vi "SynchIO.MyTest.vi"() -> ()   [LabVIEW 2016, in "SynchIO.lvclass"]
doc: "JKI State Machine Objects (SMO) 1.0.0.5\nJKI - JKI\nCopyright (c) 2016, JKI"
uses:
  SynchIO.lvclass
  C:/Program Files (x86)/National Instruments/LabVIEW 2016/vi.lib/JKI/JKI SMO/SMO/SMO.lvclass
  SynchIO.USB4431/SynchIO.USB4431.lvclass
  I:/levy_SVN/lockin/branches/jlevy/SMO/SynchIO/SynchIO.lvclass
  <vilib>/JKI/JKI SMO/SMO/Typedefs/SMOState --Enum.ctl
  <vilib>/JKI/JKI SMO/SMO/SMO.lvclass
panel:
  out "Input Signals":waveform(dbl)[](array[waveform])
  in  "4431?":bool=TRUE
  in  "IO Info":T1={"AI task"=["ai", ""], "sampling info"={"Fs"=1000.0, "#s"=1000.0}, "AO Array"=[], "AO Task"=["ao"], "Reset"=FALSE} {"sampling info"."Fs" format="%.2p"}
  out "Old Value":string
  out "New Value":string
  in  "Send":bool
  in  "Data":string
  out "error out":errorcluster
  in  "Stop":bool
  # "For instructions on how to use the JKI State Machine Objects, examples and video tutorials, visit:\nhttp://jki.net/state-machine-objects/\n\nJKI State Machine Objects™\nhttp://jki.net/state-machine-objects/\nCopyright (C) 2005-2015, JKI <info@jki.net>\nALL RIGHTS RESERVED"
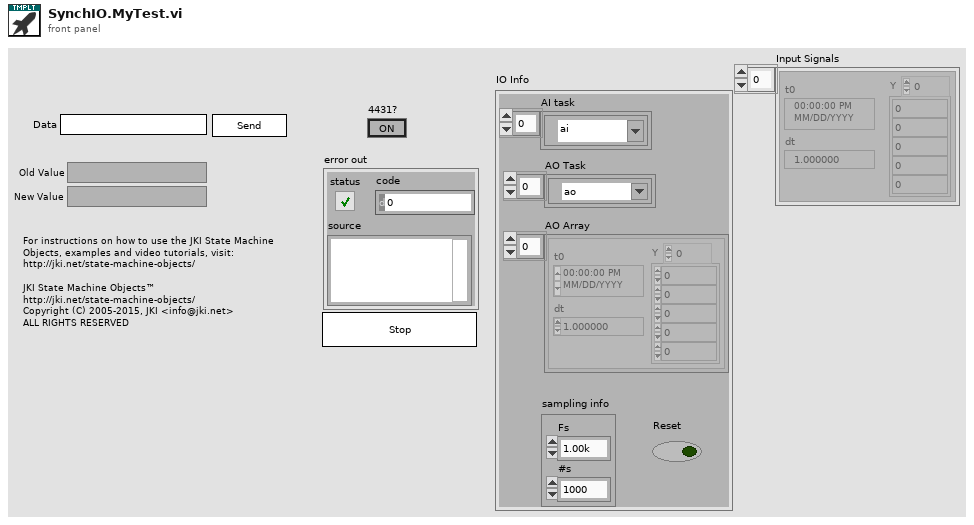
[diagram p1: front panel]
types:
  T1 = cluster{"AI task":refnum<k21>[], "sampling info":cluster{"Fs":dbl, "#s":dbl}, "AO Array":waveform(dbl)[], "AO Task":refnum<k21>[], "Reset":bool}
  T2 = typedef "SynchIO.lvclass/PublicEvents--Cluster.ctl" = cluster{"Data Changed":refnum<user-event>}
  T3 = typedef "SMO.lvclass/Public Events.ctl" = cluster{"Error":refnum<user-event>, "State":refnum<user-event>}
  T4 = cluster{"AI task":refnum<k21>[], "AO Task":refnum<k21>[]}
  T5 = typedef "SMO.lvclass/SMOState --Enum.ctl" = enum16{"unknown", "Created", "Started", "Stopped"}
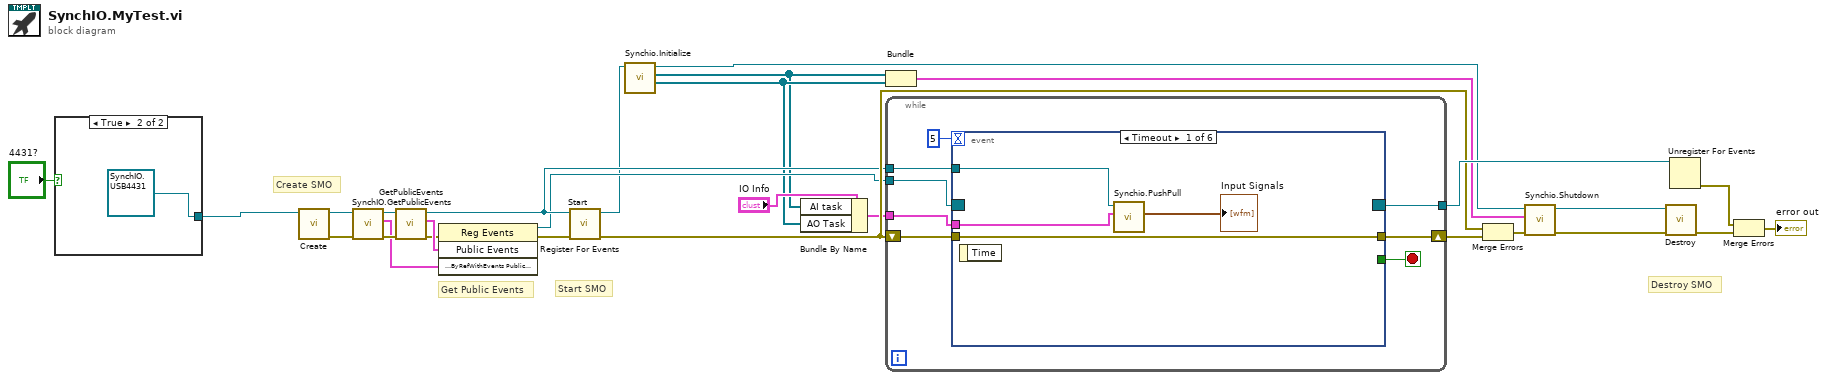
[diagram p0: block diagram]
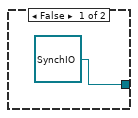
[diagram p2: hidden frame]
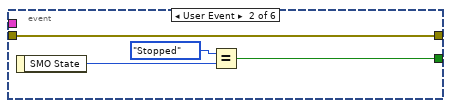
[diagram p3: hidden frame]
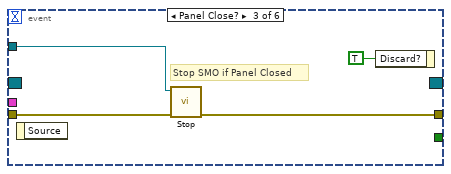
[diagram p4: hidden frame]
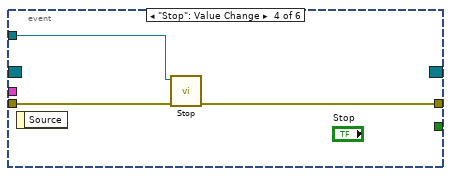
[diagram p5: hidden frame]
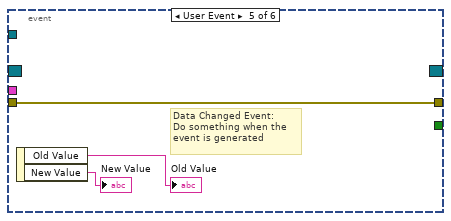
[diagram p6: hidden frame]
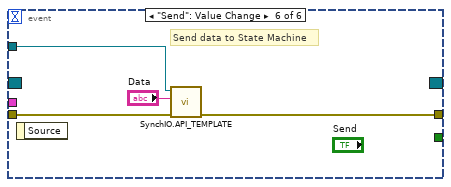
[diagram p7: hidden frame]
diagram:
  # "Get Public Events"
  # "Start SMO"
  # "Destroy SMO"
  # "Create SMO"
  n1 = case shown="True" "4431?" {
    tunnel: [refnum<class "SynchIO.lvclass"> refnum ("SMO.Template.lvclass") refnum<class "SynchIO.USB4431.lvclass"> refnum ("SynchIO.USB4431.lvclass")] -> w2
    frame False {
    }
    frame True {
    }
  }
  n2 = call <vilib>:"Create.vi"("SMO"=w2) -> ("error out"=w17:errorcluster, "SMO out"=w15:refnum<class "SynchIO.lvclass">)  [unwired: 8 in, 1 out]
  n3 = call "SynchIO.GetPublicEvents.vi"("error in (no error)"=w17, "SynchIO"=w15) -> ("error out"=w16:errorcluster, "SMO.ByRefWithEvents Public Events"=w13:T2, "SynchIO out"=w14:refnum<class "SynchIO.lvclass">)  [unwired: 7 in]
  n4 = call <vilib>:"GetPublicEvents.vi"("error in (no error)"=w16, "SMO"=w14) -> ("error out"=w19:errorcluster, "Public Events"=w20:T3, "SMO out"=w22:refnum<class "SynchIO.lvclass">)  [unwired: 7 in]
  n5 = register-events(error in=w19, w20, w13) -> (reference out=w18:refnum<event-registration>, error out=w21:errorcluster)  [unwired: 1 in]
  n6 = call <vilib>:"Start.vi"("error in (no error)"=w21, "SMO"=w22) -> ("error out"=w23:errorcluster, "SMO out"=w12:refnum<class "SynchIO.lvclass">)  [unwired: 8 in]
  n7 = call-dynamic "Synchio.Initialize.vi"("SynchIO in"=w12) -> ("AO Task"=w4:refnum<k21>[], "AI task"=w3:refnum<k21>[], "SynchIO out"=w8:refnum<class "SynchIO.lvclass">)  [unwired: 7 in, 1 out]
  n8 = Bundle By Name(cluster="IO Info", "AI task"=w3, "AO Task"=w4) -> (w10:T1)
  n9 = Bundle("AI task"=w3, "AO Task"=w4) -> (w5:T4)  [unwired: 1 in]
  n10 = while {
    shift-right: [w37] -> w27
    shift-left: w23 -> [w36]
    tunnel: w18 -> [w35]
    tunnel: [w34] -> w28
    tunnel: w22 -> [w33]
    tunnel: w10 -> [w31]
    stop <- w38 stop-if-true
    n11 = event shown="[0] Timeout" {
      selector: w35 -> [_ _ _ _ _ _]
      dyn-events: [_ _ _ _ _ _] -> w34
      timeout: 5 -> [_ _ _ _ _ _]
      tunnel: [_ w43 _ _ _ _] -> w38
      tunnel: w33 -> [w41 _ w50 w53 _ w60]
      tunnel: [w42 w46 w49 w52 w56 w57] -> w37
      tunnel: w36 -> [w42 w46 w48 w51 w56 w58]
      tunnel: w31 -> [w40 _ _ _ _ _]
      event Timeout {
        n12 = event-data() -> ()  [unwired: 1 in, 1 out]
        n13 = call-dynamic "Synchio.PushPull.vi"("IO Info"=w40, "SynchIO in"=w41) -> ("Input Signals"=→"Input Signals":waveform(dbl)[])  [unwired: 7 in, 2 out]
      }
      event User Event {
        n14 = event-data() -> ("SMO State"=w45:T5)  [unwired: 1 in]
        n15 = Equal?(x=SMOState_--Enum."Stopped", y=w45) -> (x = y?=w43:bool)
      }
      event Panel Close? {
        # "Stop SMO if Panel Closed"
        n16 = event-data() -> ()  [unwired: 1 in, 1 out]
        n17 = call <vilib>:"Stop.vi"("error in (no error)"=w48, "SMO"=w50) -> ("error out"=w49:errorcluster)  [unwired: 8 in, 1 out]
        n18 = event-data("Discard?"=TRUE ("OK")) -> ()  [unwired: 1 in, 1 out]
      }
      event "Stop": Value Change {
        n19 = event-data() -> ()  [unwired: 1 in, 1 out]
        n20 = call <vilib>:"Stop.vi"("error in (no error)"=w51, "SMO"=w53) -> ("error out"=w52:errorcluster)  [unwired: 8 in, 1 out]
      }
      event User Event {
        # "Data Changed Event:\nDo something when the\nevent is generated"
        n21 = event-data() -> ("Old Value"=→"Old Value":string, "New Value"=→"New Value":string)  [unwired: 1 in]
      }
      event "Send": Value Change {
        # "Send data to State Machine"
        n22 = event-data() -> ()  [unwired: 1 in, 1 out]
        n23 = call "SynchIO.API_TEMPLATE.vi"("error in (no error)"=w58, "myData"="Data", "SynchIO"=w60) -> ("error out"=w57:errorcluster)  [unwired: 6 in, 2 out]
      }
    }
  }
  n24 = Merge Errors(w23, w27) -> (w7:errorcluster)
  n25 = call-dynamic "Synchio.Shutdown.vi"("error in (no error)"=w7, "AIAO Tasks"=w5, "SynchIO in"=w8) -> ("error out"=w6:errorcluster, "SynchIO out"=w9:refnum<class "SynchIO.lvclass">)  [unwired: 7 in]
  n26 = call <vilib>:"Destroy.vi"("error in (no error)"=w6, "SMO"=w9) -> ("error out"=w24:errorcluster)  [unwired: 9 in]
  n27 = Unregister For Events(event registration refnum=w28) -> (error out=w26:errorcluster)  [unwired: 1 in]
  n28 = Merge Errors(w26, w24) -> (→"error out":errorcluster)
